vi "simpleCodeSandbox.vi"() -> ()   [LabVIEW 2020]
panel:
  out "Array":dbl[](array[numeric])
  out "inner block i val":i32
  in  "inner loop":i32
  out "outer block orange":dbl
  out "outer block i val":i32
  in  "OK Button":bool
  in  "outer loop":i32
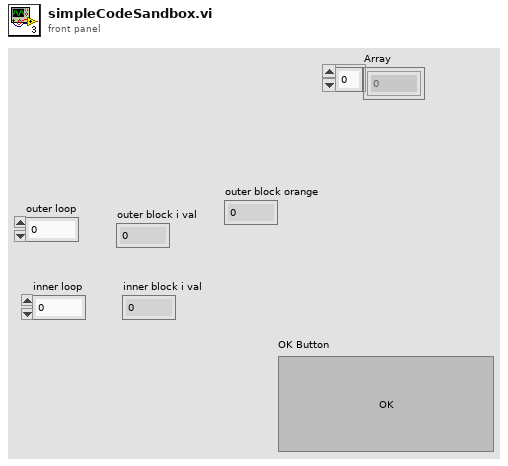
[diagram p1: front panel]
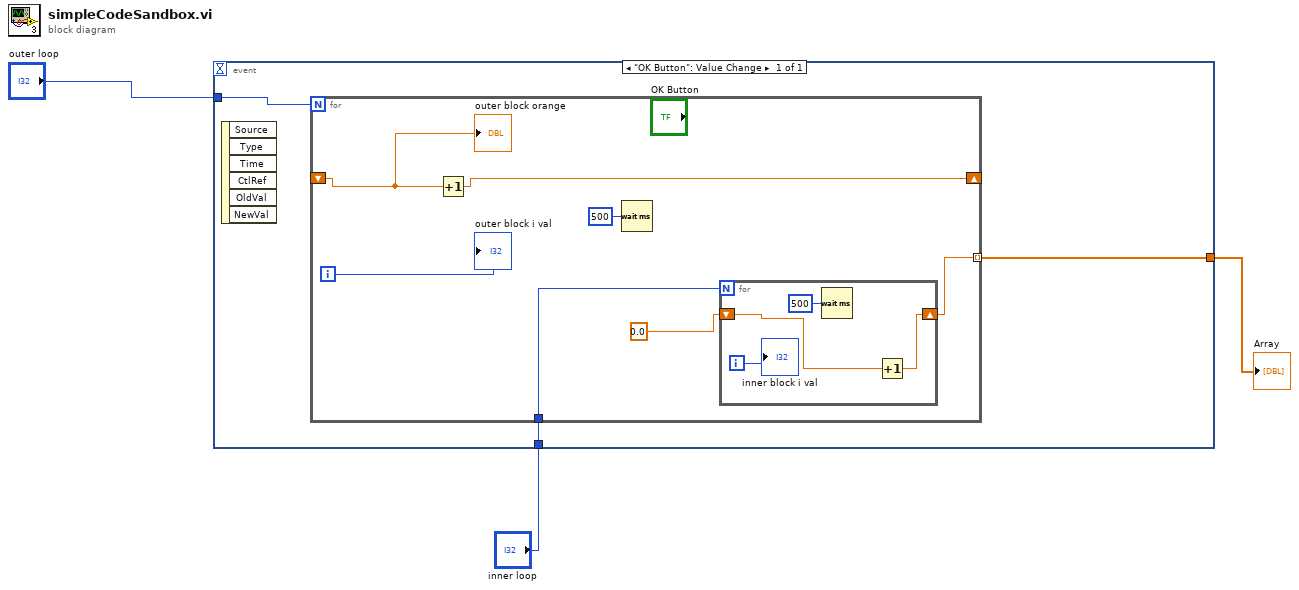
[diagram p0: block diagram]
diagram:
  n1 = event shown="[0] \"OK Button\": Value Change" {
    selector: _ -> [_]
    dyn-events: _ -> [_]
    timeout: _ -> [_]
    tunnel: "outer loop" -> [w6]
    tunnel: "inner loop" -> [w5]
    tunnel: [w4] -> w1
    event "OK Button": Value Change {
      n2 = event-data() -> ()  [unwired: 1 in, 6 out]
      n3 = for {
        N: w6 -> [_]
        shift-right: [w13] -> _
        shift-left: _ -> [w11]
        tunnel: w5 -> [w9]
        tunnel: [w8] -> w4 mode=indexing
        i -> [w12]
        n4 = Increment(x=w11) -> (x+1=w13:dbl)
        n5 = Wait (ms)(milliseconds to wait=u32 500) -> ()  [unwired: 1 out]
        n6 = for {
          N: w9 -> [_]
          shift-right: [w14] -> w8
          shift-left: 0.0 -> [w15]
          i -> [w17]
          n7 = Wait (ms)(milliseconds to wait=u32 500) -> ()  [unwired: 1 out]
          n8 = Increment(x=w15) -> (x+1=w14:dbl)
          "inner block i val" <- w17
        }
        "outer block i val" <- w12
        "outer block orange" <- w11
      }
    }
  }
  "Array" <- w1
